vi "DP_IniSigningTool.vi"() -> ()   [LabVIEW 2020]
uses:
  <vilib>/Utility/file.llb/Read Delimited Spreadsheet (string).vi
panel:
  out "?":string
  in  "GProviders files":path=path "C:/Projects/DependencyViewer/GProviders"
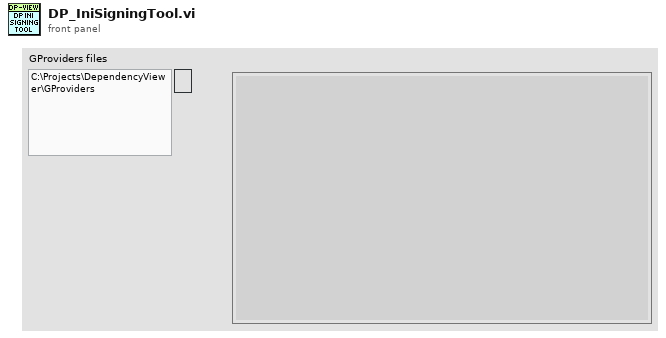
[diagram p1: front panel]
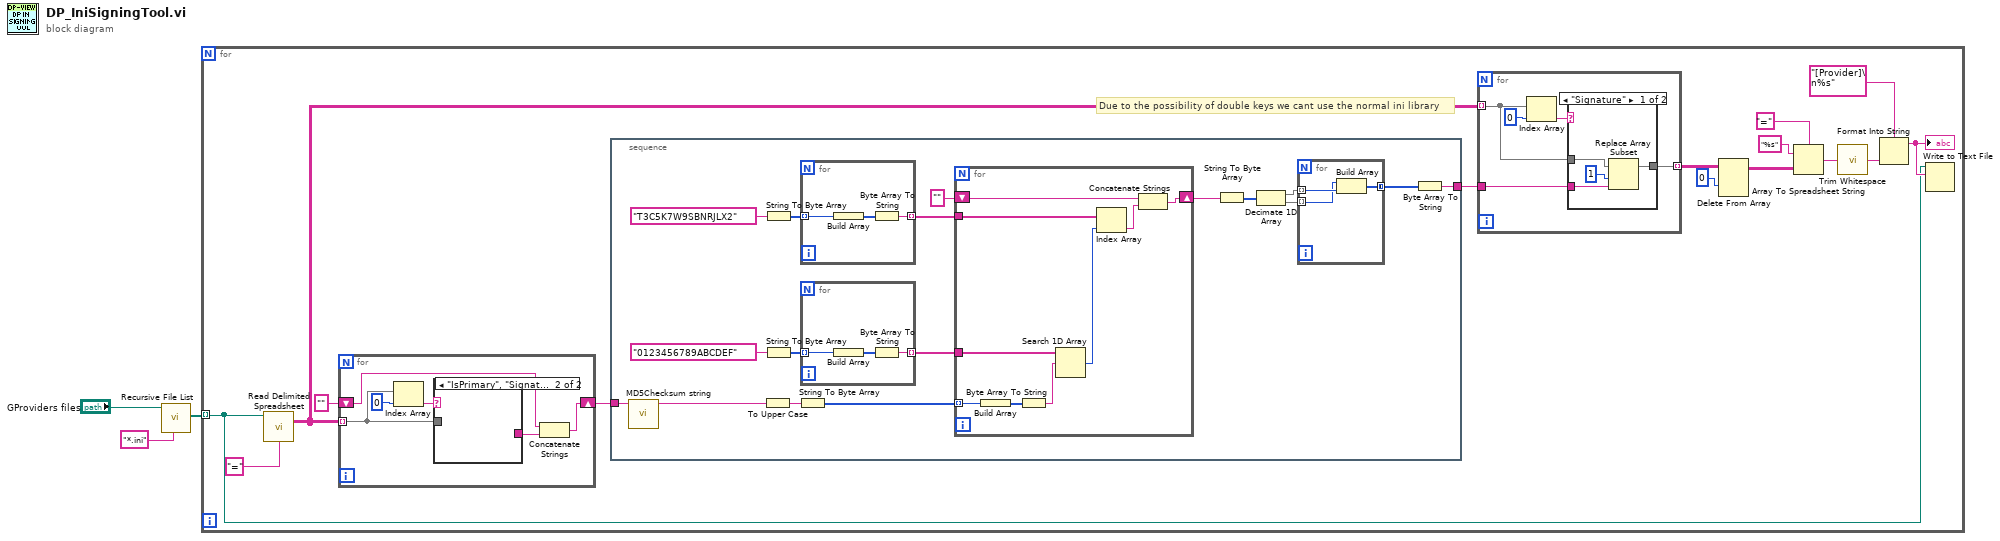
[diagram p0: block diagram]
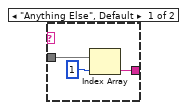
[diagram p3: hidden frame]
diagram:
  n1 = call <vilib>:"Recursive File List.vi"("pattern"="*.ini", "Folder Path"="GProviders files") -> ("All Files in Dir"=w1:path[])  [unwired: 5 in, 4 out]
  n2 = for {
    tunnel: w1 -> [w4] mode=indexing
    # "Due to the possibility of double keys we cant use the normal ini library"
    n3 = call-poly <vilib>:"Read Delimited Spreadsheet.vi"("file path (dialog if empty)"=w4, "delimiter (\\t)"="=" ("delimiter (\\t)")) -> ("all rows"=w15:string[][])  [unwired: 8 in, 5 out]
    n4 = for {
      tunnel: w15 -> [w66] mode=indexing
      shift-right: [w68] -> w16
      shift-left: "" -> [w67]
      n5 = Index Array(array=w66, index=0) -> (element=w64:string)
      n6 = case shown="\"IsPrimary\", \"Signature\"" w64 {
        tunnel: w66 -> [w71 _]
        tunnel: [w70 _] -> w65
        frame "Anything Else", Default {
          n7 = Index Array(array=w71, index=1) -> (element=w70:string)
        }
        frame "IsPrimary", "Signature" {
        }
      }
      n8 = Concatenate Strings(w67, w65) -> (w68:string)
    }
    n9 = stacked-sequence {
      tunnel: [w34] -> w14
      tunnel: w16 -> [w20]
      frame #0 {
        n10 = call <vilib>:"MD5Checksum string.vi"("Message String"=w20) -> ("MD5 message-digest"=w19:string)  [unwired: 10 in]
        n11 = To Upper Case(1:w19) -> (0:w29:string)
        n12 = String To Byte Array(string="T3C5K7W9SBNRJLX2" ("Message String")) -> (unsigned byte array=w22:u8[])
        n13 = String To Byte Array(string="0123456789ABCDEF" ("Message String")) -> (unsigned byte array=w25:u8[])
        n14 = String To Byte Array(string=w29) -> (unsigned byte array=w21:u8[])
        n15 = for {
          tunnel: w22 -> [w44] mode=indexing
          tunnel: [w42] -> w27 mode=indexing
          n16 = Build Array(w44) -> (w43:u8[])
          n17 = Byte Array To String(unsigned byte array=w43) -> (string=w42:string)
        }
        n18 = for {
          tunnel: w25 -> [w41] mode=indexing
          tunnel: [w39] -> w26 mode=indexing
          n19 = Build Array(w41) -> (w40:u8[])
          n20 = Byte Array To String(unsigned byte array=w40) -> (string=w39:string)
        }
        n21 = for {
          tunnel: w21 -> [w53] mode=indexing
          tunnel: w26 -> [w51]
          tunnel: w27 -> [w50]
          shift-right: [w48] -> w30
          shift-left: "" -> [w47]
          n22 = Build Array(w53) -> (w52:u8[])
          n23 = Byte Array To String(unsigned byte array=w52) -> (string=w45:string)
          n24 = Search 1D Array(1D array=w51, element=w45) -> (index of element=w46:i32)  [unwired: 1 in]
          n25 = Index Array(array=w50, index=w46) -> (element=w49:string)
          n26 = Concatenate Strings(w47, w49) -> (w48:string)
        }
        n27 = String To Byte Array(string=w30) -> (unsigned byte array=w35:u8[])
        n28 = Decimate 1D Array(w35) -> (w31:u8[], w32:u8[])
        n29 = for {
          tunnel: w31 -> [w38] mode=indexing
          tunnel: w32 -> [w37] mode=indexing
          tunnel: [w36] -> w33 mode=concatenating
          n30 = Build Array(w37, w38) -> (w36:u8[])
        }
        n31 = Byte Array To String(unsigned byte array=w33) -> (string=w34:string)
      }
    }
    n32 = for {
      tunnel: w15 -> [w57] mode=indexing
      tunnel: w14 -> [w55]
      tunnel: [w54] -> w13 mode=indexing
      n33 = Index Array(array=w57, index=0) -> (element=w56:string)
      n34 = case shown="\"Signature\"" w56 {
        tunnel: w57 -> [w62 w63]
        tunnel: w55 -> [w60 _]
        tunnel: [w59 w63] -> w54
        frame "Signature" {
          n35 = Replace Array Subset(array=w62, new element=w60, index=1) -> (w59:string[])
        }
        frame "Anything else", Default {
        }
      }
    }
    n36 = Delete From Array(array=w13, index (row)=0) -> (array with subset deleted=w11:string[][])  [unwired: 2 in, 1 out]
    n37 = Array To Spreadsheet String(delimiter (Tab)="=" ("delimiter (\\t)"), array=w11, 3:"%s" ("format string")) -> (spreadsheet string=w8:string)
    n38 = call <vilib>:"Trim Whitespace.vi"("string"=w8) -> ("trimmed string"=w7:string)  [unwired: 1 in]
    n39 = Format Into String(format string="[Provider]\n%s", w7) -> (resulting string=w5:string)  [unwired: 2 in, 1 out]
    "?" <- w5
    n40 = Write to Text File(file (use dialog)=w4, text=w5) -> ()  [unwired: 2 in, 3 out]
  }
